vi "PIDF.vi"(4 "reinitialize? (F)":bool, 5 "invert? (F)":bool, 6 "PIDF gains":cluster{"Kp":dbl, "Ki":dbl, "Kd":dbl, "Kf":dbl} {"Kf" format="%.3f"; "Kd" format="%.3f"; "Ki" format="%.3f"; "Kp" format="%.3f"}, 7 "output range":cluster{"output high":dbl, "output low":dbl}={"output high"=1.0, "output low"=-1.0} {"output low" format="%.2f"; "output high" format="%.2f"}, 8 "i Zone":dbl=inf format="%.2f", 9 "Feedforward":dbl, 10 "process variable":dbl format="%.2f", 11 "setpoint":dbl format="%.2f") -> (1 "In i Zone?":bool, 2 "In Range?":bool, 3 "output":dbl format="%.2f")   [LabVIEW 2017]
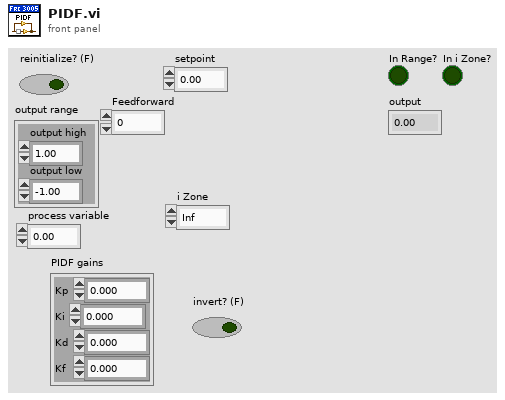
[diagram p1: front panel]
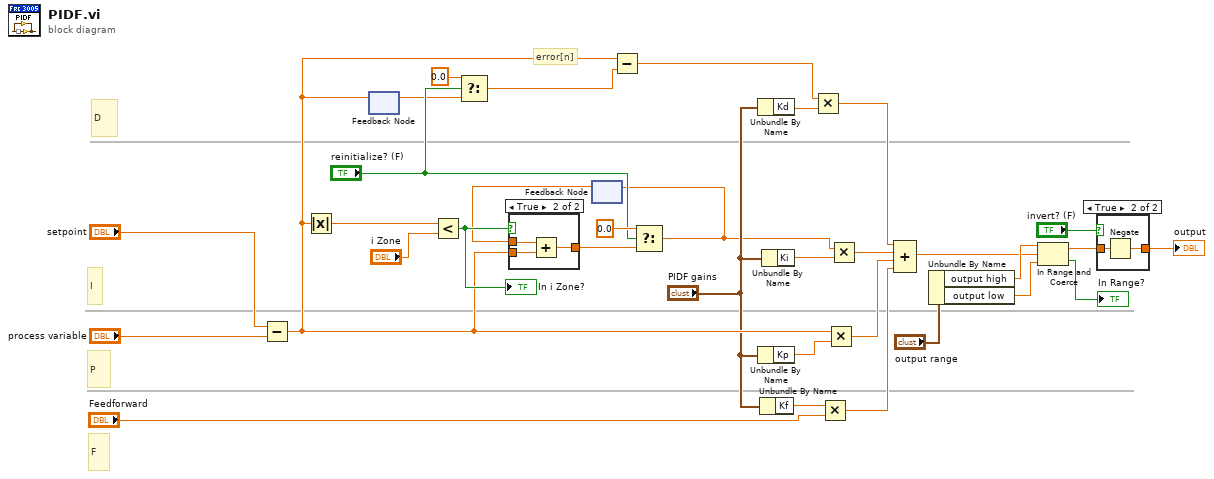
[diagram p0: block diagram]
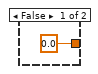
[diagram p3: hidden frame]
diagram:
  # "F"
  # "D"
  # "I"
  # "P"
  # "error[n]"
  n1 = Subtract(x="setpoint", y="process variable") -> (x-y=w24:dbl)
  n2 = Absolute Value(x=w24) -> (abs(x)=w31:dbl)
  n3 = feedback #1() -> (w22:dbl)  [unwired: 1 in]
  n4 = feedback-in #1(w24) -> ()
  n5 = Less?(x=w31, y="i Zone") -> (x < y?=w29:bool)
  "In i Zone?" <- w29
  n6 = Select(t=0.0 ("f"), s="reinitialize? (F)", f=w22) -> (s? t:f=w21:dbl)
  n7 = feedback #2() -> (w28:dbl)  [unwired: 1 in]
  n8 = case shown="True" w29 {
    tunnel: w24 -> [_ w37]
    tunnel: [0.0 ("f") w36] -> w27
    tunnel: w28 -> [_ w35]
    frame False {
    }
    frame True {
      n9 = Add(x=w35, y=w37) -> (x+y=w36:dbl)
    }
  }
  n10 = Subtract(x=w24, y=w21) -> (x-y=w11:dbl)
  n11 = Select(t=0.0 ("f"), s="reinitialize? (F)", f=w27) -> (s? t:f=w8:dbl)
  n12 = feedback-in #2(w8) -> ()
  n13 = Unbundle By Name("PIDF gains") -> ("Kd"=w12:dbl)
  n14 = Unbundle By Name("PIDF gains") -> ("Kp"=w32:dbl)
  n15 = Unbundle By Name("PIDF gains") -> ("Kf"=w14:dbl)
  n16 = Unbundle By Name("PIDF gains") -> ("Ki"=w9:dbl)
  n17 = Multiply(x=w11, y=w12) -> (x*y=w10:dbl)
  n18 = Multiply(x=w14, y="Feedforward") -> (x*y=w13:dbl)
  n19 = Multiply(x=w24, y=w32) -> (x*y=w20:dbl)
  n20 = Multiply(x=w8, y=w9) -> (x*y=w7:dbl)
  n21 = Compound Arithmetic op=ADD(w10, w7, w20, w13) -> (w16:dbl)
  n22 = Unbundle By Name("output range") -> ("output high"=w18:dbl, "output low"=w17:dbl)
  n23 = In Range and Coerce(upper limit=w18, x=w16, lower limit=w17) -> (coerced(x)=w5:dbl, In Range?=→"In Range?":bool)
  n24 = case shown="True" "invert? (F)" {
    tunnel: w5 -> [w38 w40]
    tunnel: [w38 w39] -> w4
    frame False {
    }
    frame True {
      n25 = Negate(x=w40) -> (-x=w39:dbl)
    }
  }
  "output" <- w4
